vi "weekstringmap.vi"(11 "now weekstring input":string) -> (3 "now weekstring string":string)   [LabVIEW 2011]
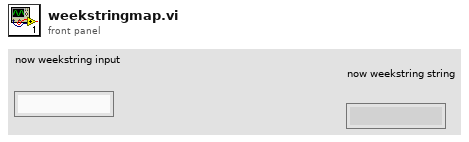
[diagram p1: front panel]
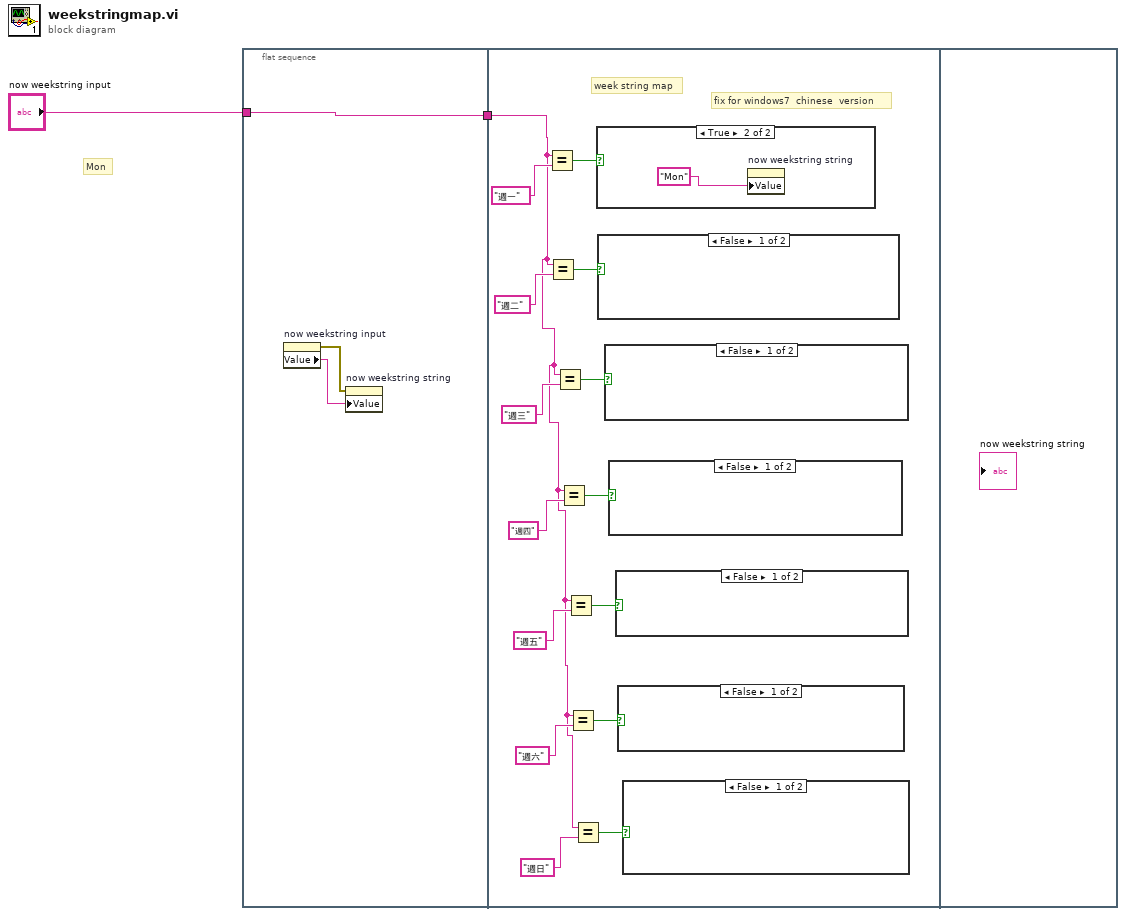
[diagram p0: block diagram]
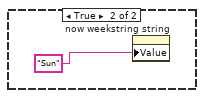
[diagram p2: hidden frame]
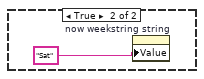
[diagram p3: hidden frame]
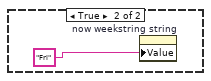
[diagram p4: hidden frame]
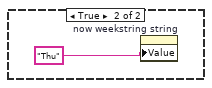
[diagram p5: hidden frame]
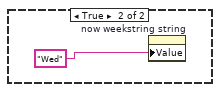
[diagram p6: hidden frame]
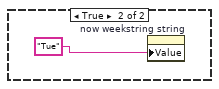
[diagram p7: hidden frame]
diagram:
  # "Mon"
  n1 = flat-sequence {
    tunnel: "now weekstring input" -> [w5]
    tunnel: [w5] -> w1
    tunnel: w1 -> [w6]
    frame #0 {
      n2 = property on="now weekstring input" class="Str"() -> (error out=w4:errorcluster, "Value"=w3:string)  [unwired: 2 in, 1 out]
      n3 = property on="now weekstring string" class="Str"(error in=w4, "Value"=w3) -> ()  [unwired: 1 in, 2 out]
    }
    frame #1 {
      # "fix for windows7  chinese  version"
      # "week string map"
      n4 = Equal?(x=w6, y="週一") -> (x = y?=w19:bool)
      n5 = Equal?(x=w6, y="週二") -> (x = y?=w17:bool)
      n6 = Equal?(x=w6, y="週三") -> (x = y?=w15:bool)
      n7 = Equal?(x=w6, y="週四") -> (x = y?=w13:bool)
      n8 = Equal?(x=w6, y="週五") -> (x = y?=w11:bool)
      n9 = Equal?(x=w6, y="週六") -> (x = y?=w9:bool)
      n10 = Equal?(x=w6, y="週日") -> (x = y?=w7:bool)
      n11 = case shown="True" w19 {
        frame False {
        }
        frame True {
          n12 = property on="now weekstring string" class="Str"("Value"="Mon") -> ()  [unwired: 2 in, 2 out]
        }
      }
      n13 = case shown="False" w17 {
        frame False {
        }
        frame True {
          n14 = property on="now weekstring string" class="Str"("Value"="Tue") -> ()  [unwired: 2 in, 2 out]
        }
      }
      n15 = case shown="False" w15 {
        frame False {
        }
        frame True {
          n16 = property on="now weekstring string" class="Str"("Value"="Wed") -> ()  [unwired: 2 in, 2 out]
        }
      }
      n17 = case shown="False" w13 {
        frame False {
        }
        frame True {
          n18 = property on="now weekstring string" class="Str"("Value"="Thu") -> ()  [unwired: 2 in, 2 out]
        }
      }
      n19 = case shown="False" w11 {
        frame False {
        }
        frame True {
          n20 = property on="now weekstring string" class="Str"("Value"="Fri") -> ()  [unwired: 2 in, 2 out]
        }
      }
      n21 = case shown="False" w9 {
        frame False {
        }
        frame True {
          n22 = property on="now weekstring string" class="Str"("Value"="Sat") -> ()  [unwired: 2 in, 2 out]
        }
      }
      n23 = case shown="False" w7 {
        frame False {
        }
        frame True {
          n24 = property on="now weekstring string" class="Str"("Value"="Sun") -> ()  [unwired: 2 in, 2 out]
        }
      }
    }
    frame #2 {
    }
  }
